vi "Android Deploy.vi"() -> ()   [LabVIEW 2016]
panel:
  in  "Constants xml":path caption="Constants File"
  in  "Host":string="172.22.11.2"
  in  "Clear Cache":bool
  in  "Clear":bool
  out "Console":string
  in  "RIOdroid Directory":path caption="RIOdroid Directory (Includes RIOdroid.tar.gz and RIOdroid.roborio.sh)"
  in  "Setup RIO":bool
  in  "Andoid APK App":path
  in  "Load APK":bool
  # "Android Vision App - Deploy Tools"
  # "Fix target failed to deploy with errors issue by clearing the object cache."
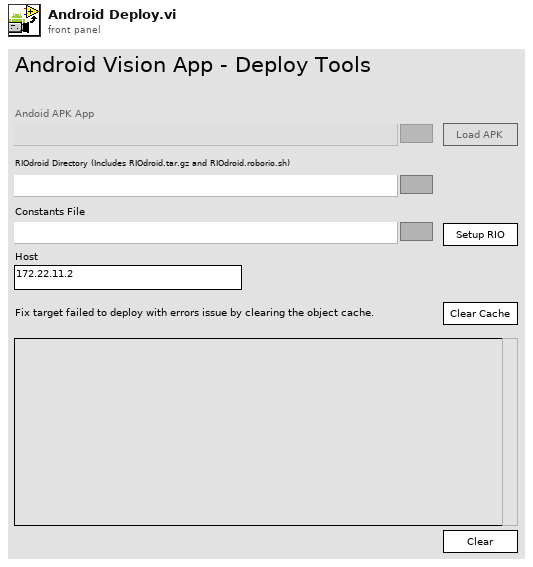
[diagram p1: front panel]
types:
  T1 = cluster{"plink":path, "pscp":path, "Console":refnum<vi>}
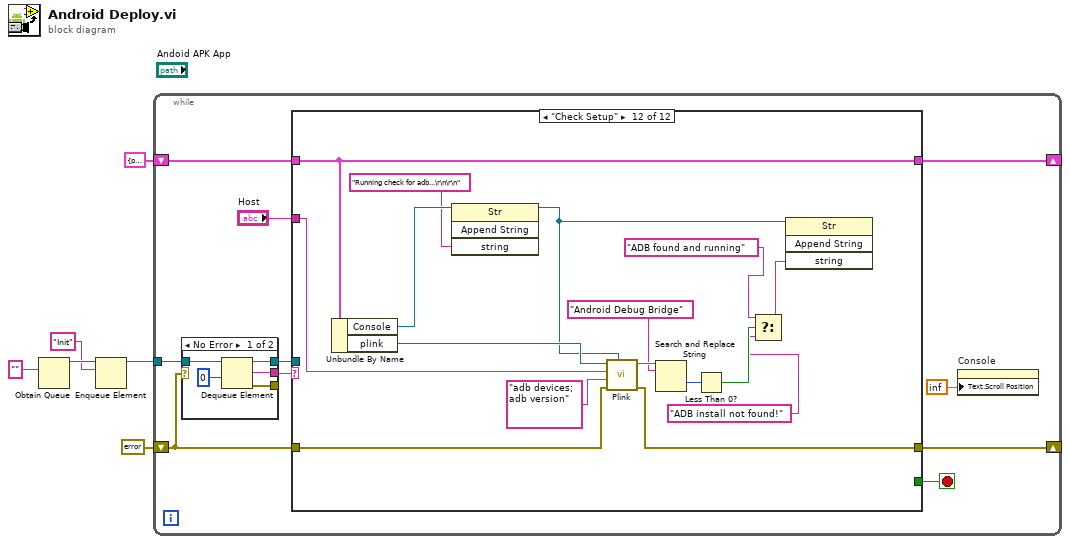
[diagram p0: block diagram]
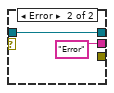
[diagram p2: hidden frame]
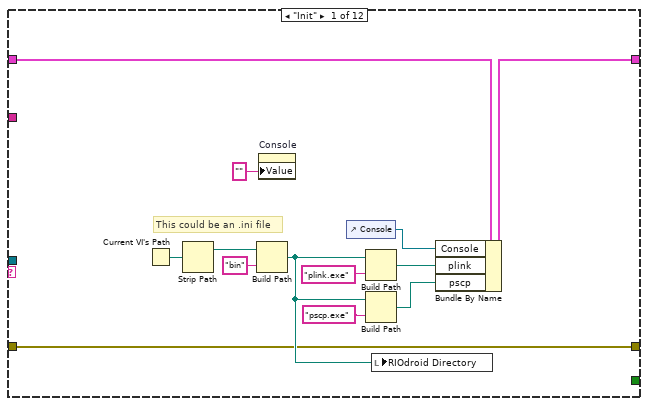
[diagram p3: hidden frame]
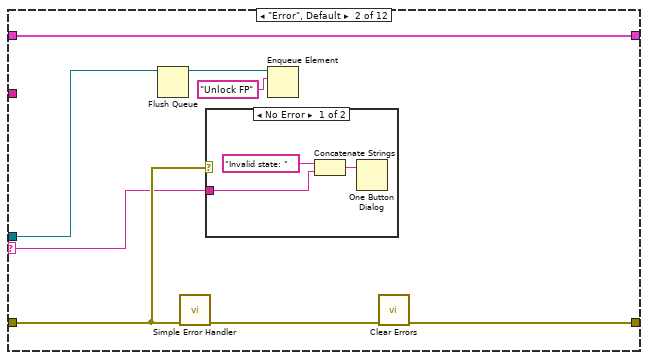
[diagram p4: hidden frame]
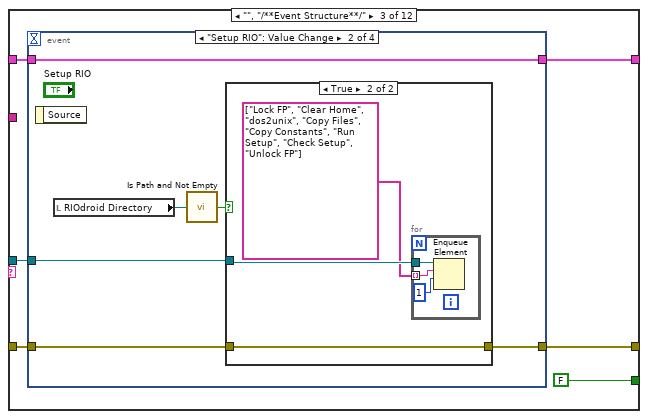
[diagram p6: hidden frame]
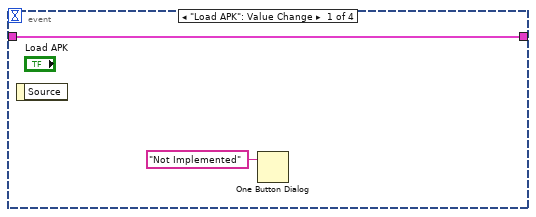
[diagram p7: hidden frame]
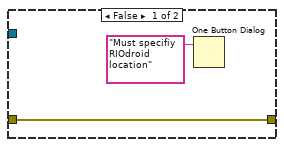
[diagram p8: hidden frame]
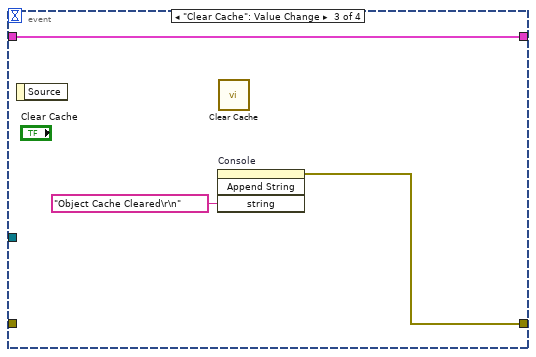
[diagram p9: hidden frame]
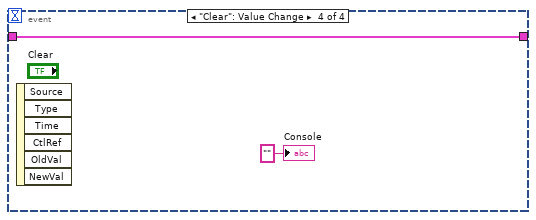
[diagram p10: hidden frame]
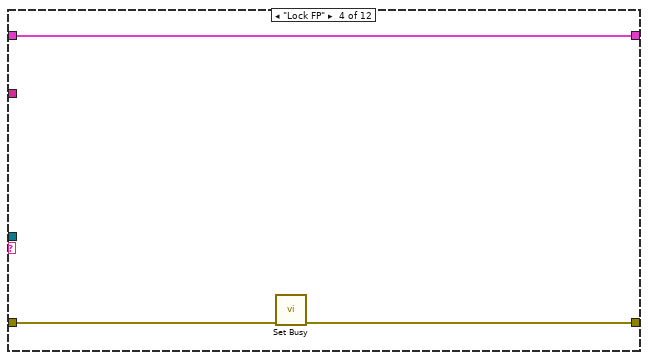
[diagram p11: hidden frame]
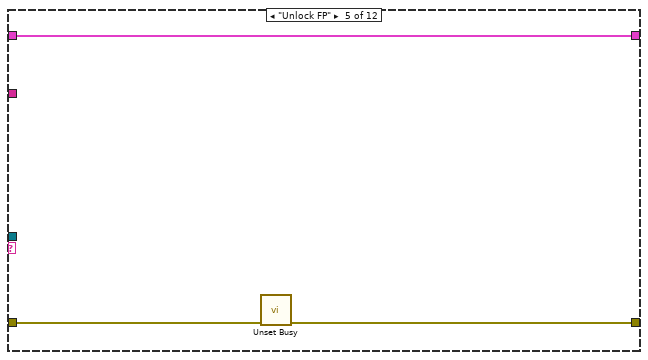
[diagram p12: hidden frame]
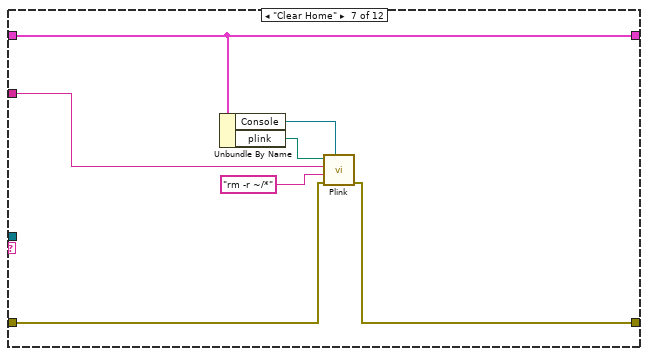
[diagram p14: hidden frame]
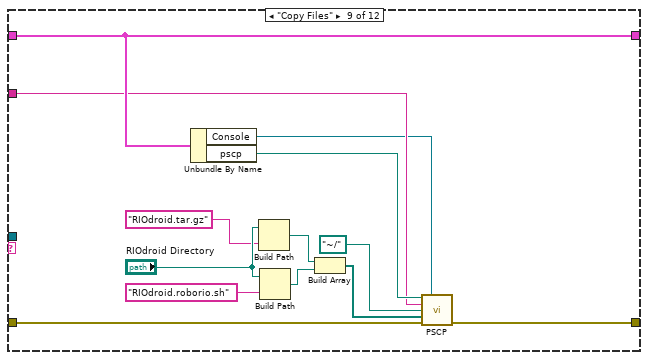
[diagram p16: hidden frame]
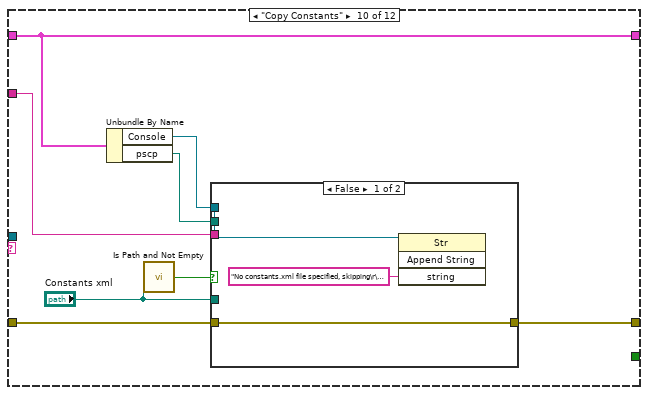
[diagram p17: hidden frame]
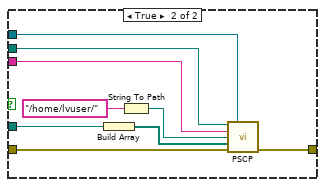
[diagram p18: hidden frame]
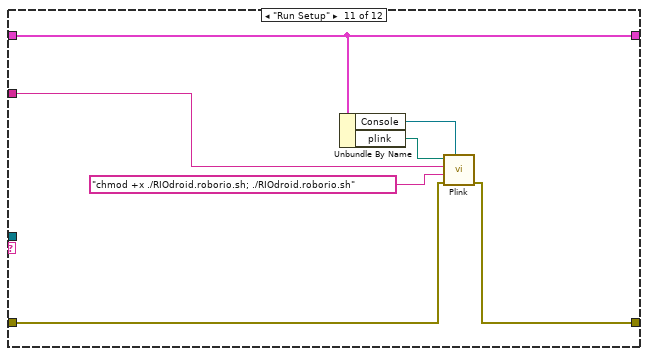
[diagram p19: hidden frame]
diagram:
  n1 = Obtain Queue(element data type="" ("Console")) -> (queue out=w5:refnum<queue>)  [unwired: 4 in, 2 out]
  n2 = Enqueue Element(queue=w5, element="Init") -> (queue out=w4:refnum<queue>)  [unwired: 2 in, 2 out]
  n3 = while {
    tunnel: w4 -> [w15]
    shift-right: [w12] -> _
    shift-left: T1 {"plink"=path "", "pscp"=path "", "Console"=refnum} -> [w13]
    shift-right: [w10] -> _
    shift-left: errorcluster {"status"=FALSE, "code"=0, "source"=""} ("error out") -> [w7]
    stop <- w14 stop-if-true
    n4 = case shown="No Error" w7 {
      tunnel: [w21 "Error" ("Console")] -> w16
      tunnel: w15 -> [w20 w23]
      tunnel: [w18 w23] -> w8
      tunnel: [w17 _] -> _
      frame No Error {
        n5 = Dequeue Element(queue=w20, timeout in ms (-1)=0) -> (queue out=w18:refnum<queue>, element=w21:string, error out=w17:errorcluster)  [unwired: 1 in, 1 out]
      }
      frame Error {
      }
    }
    n6 = case shown="\"Check Setup\"" w16 {
      selector: w16 -> [_ w40 _ _ _ _ _ _ _ _ _ _]
      tunnel: [_ _ FALSE _ _ _ _ _ _ _ _ _] -> w14
      tunnel: [w24 w42 w48 w75 w78 w81 w84 w90 w103 w111 w126 w142] -> w10
      tunnel: w13 -> [w30 w44 w52 w77 w80 w82 w87 w91 w100 w110 w129 w145]
      tunnel: [w29 w44 w51 w77 w80 w82 w87 w91 w100 w110 w129 w145] -> w12
      tunnel: "Host" -> [_ _ _ _ _ _ w88 _ w98 w108 w130 w146]
      tunnel: w7 -> [w24 w41 w49 w76 w79 w81 w85 w90 w104 w112 w127 w143]
      tunnel: w8 -> [_ w39 w50 _ _ _ _ _ _ _ _ _]
      frame "Init" {
        # "This could be an .ini file"
        n7 = Current VI's Path() -> (path=w31:path)
        n8 = Strip Path(path=w31) -> (stripped path=w32:path)  [unwired: 1 out]
        n9 = Build Path(base path=w32, name or relative path="bin") -> (appended path=w28:path)
        n10 = property on="Console" class="Str"("Value"="" ("Console")) -> ()  [unwired: 2 in, 2 out]
        n11 = control-ref of="Console"() -> (w25:refnum<vi>)
        n12 = Build Path(base path=w28, name or relative path="plink.exe") -> (appended path=w26:path)
        n13 = Build Path(base path=w28, name or relative path="pscp.exe") -> (appended path=w27:path)
        n14 = local write "RIOdroid Directory"(w28) -> ()
        n15 = Bundle By Name(cluster=w30, "Console"=w25, "plink"=w26, "pscp"=w27) -> (w29:T1)
      }
      frame "Error", Default {
        n16 = Flush Queue(queue=w39) -> (queue out=w38:refnum<queue>)  [unwired: 1 in, 2 out]
        n17 = call <vilib>:"Simple Error Handler.vi"("error in (no error)"=w41) -> ("error out"=w43:errorcluster)  [unwired: 4 in, 4 out]
        n18 = case shown="No Error" w41 {
          tunnel: w40 -> [w46 _]
          frame No Error {
            n19 = Concatenate Strings("Invalid state: " ("message"), w46) -> (w45:string)
            n20 = One Button Dialog(message=w45) -> ()  [unwired: 1 in, 1 out]
          }
          frame Error {
          }
        }
        n21 = Enqueue Element(queue=w38, element="Unlock FP") -> ()  [unwired: 2 in, 3 out]
        n22 = call <vilib>:"Clear Errors.vi"("error in (no error)"=w43) -> ("error out"=w42:errorcluster)  [unwired: 5 in, 1 out]
      }
      frame "", "/**Event Structure**/" {
        n23 = event shown="[1] \"Setup RIO\": Value Change" {
          selector: _ -> [_ _ _ _]
          dyn-events: _ -> [_ _ _ _]
          timeout: _ -> [_ _ _ _]
          tunnel: w52 -> [w55 w61 w71 w73]
          tunnel: [w55 w61 w71 w73] -> w51
          tunnel: w50 -> [_ w56 _ _]
          tunnel: w49 -> [_ w59 _ _]
          tunnel: [_ w58 w70 _] -> w48
          event "Load APK": Value Change {
            n24 = event-data() -> ()  [unwired: 1 in, 1 out]
            n25 = One Button Dialog(message="Not Implemented") -> ()  [unwired: 1 in, 1 out]
          }
          event "Setup RIO": Value Change {
            n26 = event-data() -> ()  [unwired: 1 in, 1 out]
            n27 = local read "RIOdroid Directory"() -> (w60:path)
            n28 = call <vilib>:"Is Path and Not Empty.vi"("path"=w60) -> ("Is Path and Not Empty?"=w57:bool)  [unwired: 4 in]
            n29 = case shown="True" w57 {
              tunnel: w59 -> [w63 w66]
              tunnel: [w63 w66] -> w58
              tunnel: w56 -> [_ w65]
              frame False {
                n30 = One Button Dialog(message="Must specifiy RIOdroid location") -> ()  [unwired: 1 in, 1 out]
              }
              frame True {
                n31 = for {
                  tunnel: w65 -> [w69]
                  tunnel: string[] ["Lock FP", "Clear Home", "dos2unix", "Copy Files", "Copy Constants", "Run Setup", "Check Setup", "Unlock FP"] -> [w68] mode=indexing
                  n32 = Enqueue Element(queue=w69, element=w68, timeout in ms (-1)=1) -> ()  [unwired: 1 in, 3 out]
                }
              }
            }
          }
          event "Clear Cache": Value Change {
            n33 = event-data() -> ()  [unwired: 1 in, 1 out]
            n34 = invoke on="Console" class="Str" method="Append String"("string"="Object Cache Cleared\r\n") -> (error out=w70:errorcluster)  [unwired: 3 in, 3 out]
            n35 = call "Clear Cache.vi"() -> ()  [unwired: 12 in]
          }
          event "Clear": Value Change {
            n36 = event-data() -> ()  [unwired: 1 in, 6 out]
            "Console" <- "" ("Console")
          }
        }
      }
      frame "Lock FP" {
        n37 = call <vilib>:"Set Busy.vi"("error in (no error)"=w76) -> ("error out"=w75:errorcluster)  [unwired: 9 in, 1 out]
      }
      frame "Unlock FP" {
        n38 = call <vilib>:"Unset Busy.vi"("error in (no error)"=w79) -> ("error out"=w78:errorcluster)  [unwired: 10 in]
      }
      frame "/**Setup RIO States**/" {
      }
      frame "Clear Home" {
        n39 = Unbundle By Name(w87) -> ("Console"=w83:refnum<vi>, "plink"=w86:path)
        n40 = call "Plink.vi"("Console"=w83, "error in"=w85, "Command(s) to Execute"="rm -r ~/*", "Host"=w88, "plink path"=w86) -> ("error out"=w84:errorcluster)  [unwired: 2 in, 4 out]
      }
      frame "dos2unix" {
        # "Convert any text file from dos line endings to unix before sending"
      }
      frame "Copy Files" {
        n41 = Unbundle By Name(w100) -> ("Console"=w92:refnum<vi>, "pscp"=w99:path)
        n42 = Build Path(base path="RIOdroid Directory", name or relative path="RIOdroid.tar.gz") -> (appended path=w94:path)
        n43 = Build Path(base path="RIOdroid Directory", name or relative path="RIOdroid.roborio.sh") -> (appended path=w102:path)
        n44 = Build Array(w94, w102) -> (w97:path[])
        n45 = call "PSCP.vi"("pscp path"=w99, "Console"=w92, "Host"=w98, "remote path"=path "~/", "Files"=w97, "error in"=w104) -> ("error out"=w103:errorcluster)  [unwired: 5 in, 4 out]
      }
      frame "Copy Constants" {
        n46 = Unbundle By Name(w110) -> ("Console"=w107:refnum<vi>, "pscp"=w109:path)
        n47 = call <vilib>:"Is Path and Not Empty.vi"("path"="Constants xml") -> ("Is Path and Not Empty?"=w106:bool)  [unwired: 4 in]
        n48 = case shown="False" w106 {
          tunnel: w112 -> [w115 w124]
          tunnel: [w115 w123] -> w111
          tunnel: w109 -> [_ w122]
          tunnel: w108 -> [_ w121]
          tunnel: w107 -> [w114 w119]
          tunnel: "Constants xml" -> [_ w118]
          frame False {
            n49 = invoke class="Str" method="Append String"(reference=w114, "string"="No constants.xml file specified, skipping\r\n\r\n") -> ()  [unwired: 2 in, 4 out]
          }
          frame True {
            n50 = Build Array(w118) -> (w120:path[])
            n51 = String To Path(string="/home/lvuser/") -> (path=w116:path)
            n52 = call "PSCP.vi"("pscp path"=w122, "Console"=w119, "Host"=w121, "remote path"=w116, "Files"=w120, "error in"=w124) -> ("error out"=w123:errorcluster)  [unwired: 5 in, 4 out]
          }
        }
      }
      frame "Run Setup" {
        n53 = Unbundle By Name(w129) -> ("Console"=w125:refnum<vi>, "plink"=w128:path)
        n54 = call "Plink.vi"("Console"=w125, "error in"=w127, "Command(s) to Execute"="chmod +x ./RIOdroid.roborio.sh; ./RIOdroid.roborio.sh", "Host"=w130, "plink path"=w128) -> ("error out"=w126:errorcluster)  [unwired: 2 in, 4 out]
      }
      frame "Check Setup" {
        n55 = Unbundle By Name(w145) -> ("Console"=w141:refnum<vi>, "plink"=w144:path)
        n56 = invoke class="Str" method="Append String"(reference=w141, "string"="Running check for adb...\r\n\r\n") -> (reference out=w132:refnum<vi>)  [unwired: 2 in, 3 out]
        n57 = call "Plink.vi"("Console"=w132, "error in"=w143, "Command(s) to Execute"="adb devices; adb version", "Host"=w146, "plink path"=w144) -> ("error out"=w142:errorcluster, "Command Return Value(s)"=w139:string)  [unwired: 2 in, 3 out]
        n58 = Search and Replace String(input string=w139, search string="Android Debug Bridge") -> (offset past replacement=w137:i32)  [unwired: 6 in, 3 out]
        n59 = Less Than 0?(x=w137) -> (x < 0?=w136:bool)
        n60 = Select(t="ADB found and running" ("search string"), s=w136, f="ADB install not found!" ("search string")) -> (s? t:f=w133:string)
        n61 = invoke class="Str" method="Append String"(reference=w132, "string"=w133) -> ()  [unwired: 2 in, 4 out]
      }
    }
    n62 = property on="Console" class="Str"("Text.Scroll Position"=inf) -> ()  [unwired: 2 in, 2 out]
  }
